vi "S2C_VLFT10_Proc_WaitForRebootReset.vi"(8 "Error In":errorcluster) -> (0 "Error Out":errorcluster, 3 "Result":string)   [LabVIEW 2015]
uses:
  Fornax/VIs/PolyDriver/Typedefs/ExternalCommCommand.ctl
  Fornax/VIs/PolyDriver/S2C_FORNAX_Poly_CloseFornax.vi
  Fornax/VIs/PolyDriver/S2C_FORNAX_Poly_ExternalCommCommand.vi
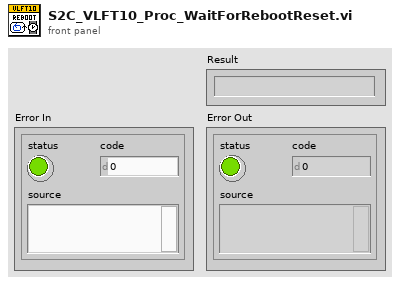
[diagram p1: front panel]
types:
  T1 = cluster{"PostDelay (ms)":i32, "ClearFornaxMsgs":bool}
  T2 = typedef "ExternalCommCommand.ctl" = i16
  T3 = cluster{"Partition":string, "Message":string, "M_CommandOptions":string, "M_ControllerBoardId":string, "M_ClientId":string, "M_Command":T2}
  T4 = cluster{"Driver":string, "Command":string, "Return":string, "Parameters":string, "Timeout":dbl}
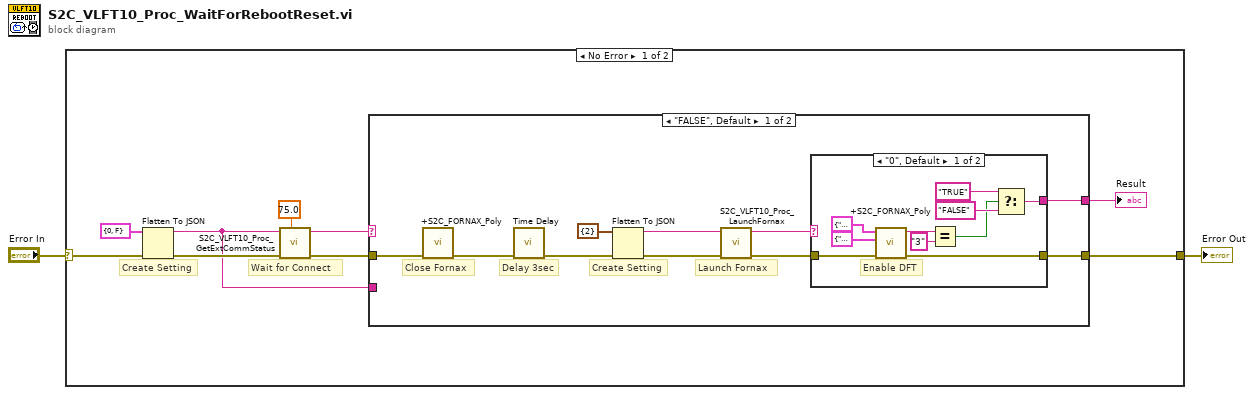
[diagram p0: block diagram]
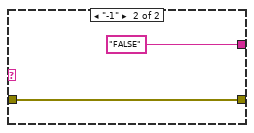
[diagram p2: hidden frame]
diagram:
  n1 = case shown="No Error" "Error In" {
    selector: "Error In" -> [w11 w36]
    tunnel: [w4 w36] -> w1
    frame No Error {
      # "Wait for Connect"
      # "Create Setting"
      n2 = Flatten To JSON(anything=T1 {"PostDelay (ms)"=0, "ClearFornaxMsgs"=FALSE}, error in (no error)=w11) -> (JSON string=w5:string, 11:w9:errorcluster)  [unwired: 1 in]
      n3 = call "S2C_VLFT10_Proc_GetExtCommStatus.vi"("Timeout"=75.0, "Error In"=w9, "Status"=w5) -> ("Error Out"=w7:errorcluster, "Result"=w6:string)  [unwired: 7 in]
      n4 = case shown="\"FALSE\", Default" w6 {
        selector: w6 -> [_ w35]
        tunnel: w7 -> [w21 w34]
        tunnel: w5 -> [_ _]
        tunnel: [w12 w34] -> w4
        tunnel: [w13 w35] -> w3
        frame "FALSE", Default {
          # "Launch Fornax"
          # "Create Setting"
          # "Delay 3sec"
          # "Close Fornax"
          n5 = call-poly "+S2C_FORNAX_Poly.vi"("Error In"=w21) -> ("Error Out"=w20:errorcluster)  [unwired: 9 in, 1 out]
          n6 = call "Time Delay"("error in (no error)"=w20) -> ("error out"=w19:errorcluster)  [unwired: 10 in]
          n7 = Flatten To JSON(anything=cluster{"Selection":u16} {"Selection"=2}, error in (no error)=w19) -> (JSON string=w16:string, 11:w17:errorcluster)  [unwired: 1 in]
          n8 = call "S2C_VLFT10_Proc_LaunchFornax.vi"("Error In"=w17, "Selection"=w16) -> ("Error Out"=w15:errorcluster, "Version"=w14:string)  [unwired: 8 in]
          n9 = case shown="\"0\", Default" w14 {
            tunnel: w15 -> [w29 w32]
            tunnel: [w25 "FALSE"] -> w13
            tunnel: [w28 w32] -> w12
            frame "0", Default {
              # "Enable DFT"
              n10 = call-poly "+S2C_FORNAX_Poly.vi"("Error In"=w29, "ExternalCommCommand"=T3 {"Partition"="Default", "Message"="ExternalCommCommand", "M_CommandOptions"="", "M_ControllerBoardId"="", "M_ClientId"="", "M_Command"=5}, "Settings"=T4 {"Driver"="Fornax", "Command"="ExternalCommCommand", "Return"="M_DftMode", "Parameters"="", "Timeout"=10.0}) -> ("Error Out"=w28:errorcluster, "Response"=w24:string)  [unwired: 7 in]
              n11 = Equal?(x=w24, y="3") -> (x = y?=w22:bool)
              n12 = Select(t="TRUE", s=w22, f="FALSE") -> (s? t:f=w25:string)
            }
            frame "-1" {
            }
          }
        }
        frame "TRUE" {
        }
      }
      "Result" <- w3
    }
    frame Error {
    }
  }
  "Error Out" <- w1
